vi "Get Output Channel Registers.vi"(8 "error in (no error)":errorcluster, 11 "Output Channels":T3[](array[typedef]) format="%.0x") -> (0 "error out":errorcluster, 3 "Output Register Info":T2(array[cluster]))   [LabVIEW 2010, in "Sensor Simulation Custom Device.lvlib"]
uses:
  Sensor Simulation Custom Device.lvlib
  <vilib>/NI Veristand/Custom Device API/Custom Device Item Ref.ctl
  TypeDefs/OutputChannelTypes.ctl
  <vilib>/NI Veristand/Custom Device API/Custom Device API.lvlib
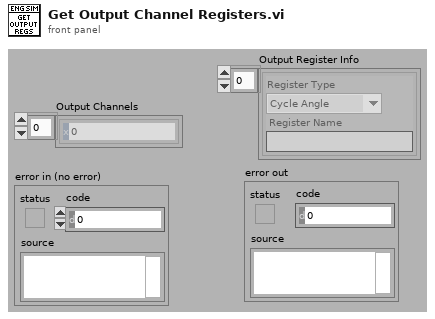
[diagram p1: front panel]
types:
  T1 = typedef "Sensor Simulation Custom Device.lvlib/OutputChannelTypes.ctl" = enum16{"Cycle Angle", "Crank Angle", "Time Duration", "Angle Duration", "Start Angle", "End Angle"}
  T2 = cluster{"Register Type":T1, "Register Name":string}[]
  T3 = typedef "Custom Device API.lvlib/Custom Device Item Ref.ctl" = u64
  T4 = typedef "Custom Device API.lvlib/Custom Device Item Info.ctl" = cluster{"Name":string, "Is Channel":bool, "GUID":string}
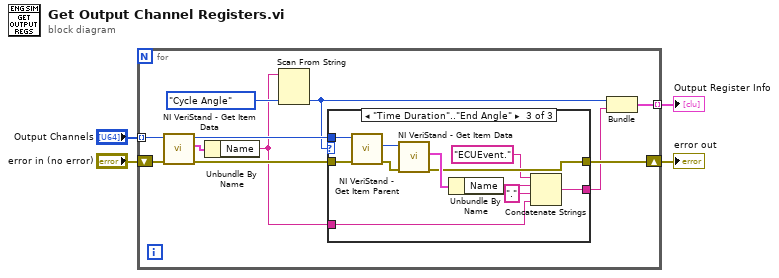
[diagram p0: block diagram]
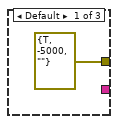
[diagram p2: hidden frame]
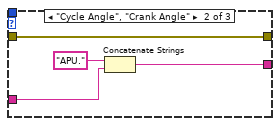
[diagram p3: hidden frame]
diagram:
  n1 = for {
    tunnel: "Output Channels" -> [w15] mode=indexing
    shift-right: [w10] -> w4
    shift-left: "error in (no error)" -> [w11]
    tunnel: [w6] -> w1 mode=indexing
    n2 = call <vilib>:"NI VeriStand - Get Item Data.vi"("error in (no error)"=w11, "Item Ref in"=w15) -> ("error out"=w12:errorcluster, "Item Info"=w14:T4, "Item Ref out"=w13:T3)  [unwired: 6 in, 1 out]
    n3 = Unbundle By Name(w14) -> ("Name"=w8:string)
    n4 = Scan From String(input string=w8, default 1=OutputChannelTypes."Cycle Angle" ("Output Channel Types")) -> (output 1=w7:T1)  [unwired: 3 in, 3 out]
    n5 = case shown="\"Time Duration\"..\"End Angle\"" w7 {
      tunnel: w13 -> [_ _ w31]
      tunnel: w12 -> [_ w18 w30]
      tunnel: [errorcluster {"status"=TRUE, "code"=-5000, "source"=""} ("error out") w18 w28] -> w10
      tunnel: [_ w19 w25] -> w5
      tunnel: w8 -> [_ w17 w24]
      frame Default {
      }
      frame "Cycle Angle", "Crank Angle" {
        n6 = Concatenate Strings("APU." ("string"), w17) -> (w19:string)
      }
      frame "Time Duration".."End Angle" {
        n7 = call <vilib>:"NI VeriStand - Get Item Parent.vi"("error in (no error)"=w30, "Item Ref in"=w31) -> ("error out"=w21:errorcluster, "Parent Ref"=w22:T3)  [unwired: 6 in, 2 out]
        n8 = call <vilib>:"NI VeriStand - Get Item Data.vi"("error in (no error)"=w21, "Item Ref in"=w22) -> ("error out"=w28:errorcluster, "Item Info"=w29:T4)  [unwired: 6 in, 2 out]
        n9 = Unbundle By Name(w29) -> ("Name"=w23:string)
        n10 = Concatenate Strings("ECUEvent." ("string"), w23, "." ("string"), w24) -> (w25:string)
      }
    }
    n11 = Bundle("Output Channel Types"=w7, w5) -> (w6:cluster{"Output Channel Types":T1, string})  [unwired: 1 in]
  }
  "error out" <- w4
  "Output Register Info" <- w1
